vi "SeCrTS-DD signal names extracter.vi"(11 "input cluster":T1) -> (3 "Signal names":T2)   [LabVIEW 2022 SP3]
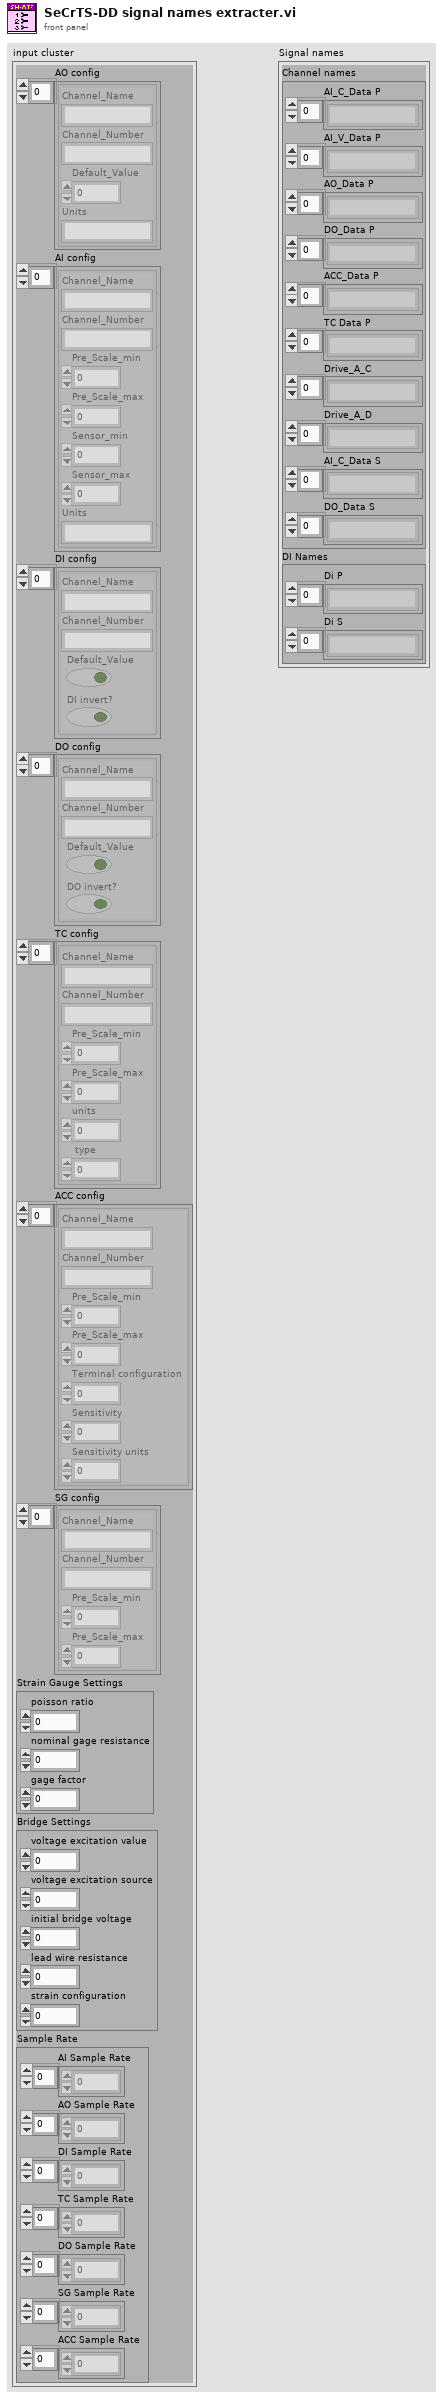
[diagram p1: front panel]
types:
  T1 = cluster{"AO config":cluster{"Channel_Name":string, "Channel_Number":string, "Default_Value":dbl, "Units":string}[], "AI config":cluster{"Channel_Name":string, "Channel_Number":string, "Pre_Scale_min":dbl, "Pre_Scale_max":dbl, "Sensor_min":dbl, "Sensor_max":dbl, "Units":string}[], "DI config":cluster{"Channel_Name":string, "Channel_Number":string, "Default_Value":bool, "DI invert?":bool}[], "DO config":cluster{"Channel_Name":string, "Channel_Number":string, "Default_Value":bool, "DO invert?":bool}[], "TC config":cluster{"Channel_Name":string, "Channel_Number":string, "Pre_Scale_min":dbl, "Pre_Scale_max":dbl, "units":i32, " type":i32}[], "ACC config":cluster{"Channel_Name":string, "Channel_Number":string, "Pre_Scale_min":dbl, "Pre_Scale_max":dbl, "Terminal configuration":i32, "Sensitivity":dbl, "Sensitivity units":i32}[], "SG config":cluster{"Channel_Name":string, "Channel_Number":string, "Pre_Scale_min":dbl, "Pre_Scale_max":dbl}[], "Strain Gauge Settings":cluster{"poisson ratio":dbl, "nominal gage resistance":dbl, "gage factor":dbl}, "Bridge Settings":cluster{"voltage excitation value":dbl, "voltage excitation source":i32, "initial bridge voltage":dbl, "lead wire resistance":dbl, "strain configuration":i32}, "Sample Rate":cluster{"AI Sample Rate":dbl[], "AO Sample Rate":dbl[], "DI Sample Rate":dbl[], "TC Sample Rate":dbl[], "DO Sample Rate":dbl[], "SG Sample Rate":dbl[], "ACC Sample Rate":dbl[]}}
  T2 = cluster{"Channel names":cluster{"AI_C_Data P":string[], "AI_V_Data P":string[], "AO_Data P":string[], "DO_Data P":string[], "ACC_Data P":string[], "TC Data P":string[], "Drive_A_C":string[], "Drive_A_D":string[], "AI_C_Data S":string[], "DO_Data S":string[]}, "DI Names":cluster{"Di P":string[], "Di S":string[]}}
  T3 = cluster{"Channel_Name":string, "Channel_Number":string, "Default_Value":dbl, "Units":string}[]
  T4 = cluster{"Channel_Name":string, "Channel_Number":string, "Pre_Scale_min":dbl, "Pre_Scale_max":dbl, "Sensor_min":dbl, "Sensor_max":dbl, "Units":string}[]
  T5 = cluster{"Channel_Name":string, "Channel_Number":string, "Default_Value":bool, "DI invert?":bool}[]
  T6 = cluster{"Channel_Name":string, "Channel_Number":string, "Default_Value":bool, "DO invert?":bool}[]
  T7 = cluster{"Channel_Name":string, "Channel_Number":string, "Pre_Scale_min":dbl, "Pre_Scale_max":dbl, "units":i32, " type":i32}[]
  T8 = cluster{"Channel_Name":string, "Channel_Number":string, "Pre_Scale_min":dbl, "Pre_Scale_max":dbl, "Terminal configuration":i32, "Sensitivity":dbl, "Sensitivity units":i32}[]
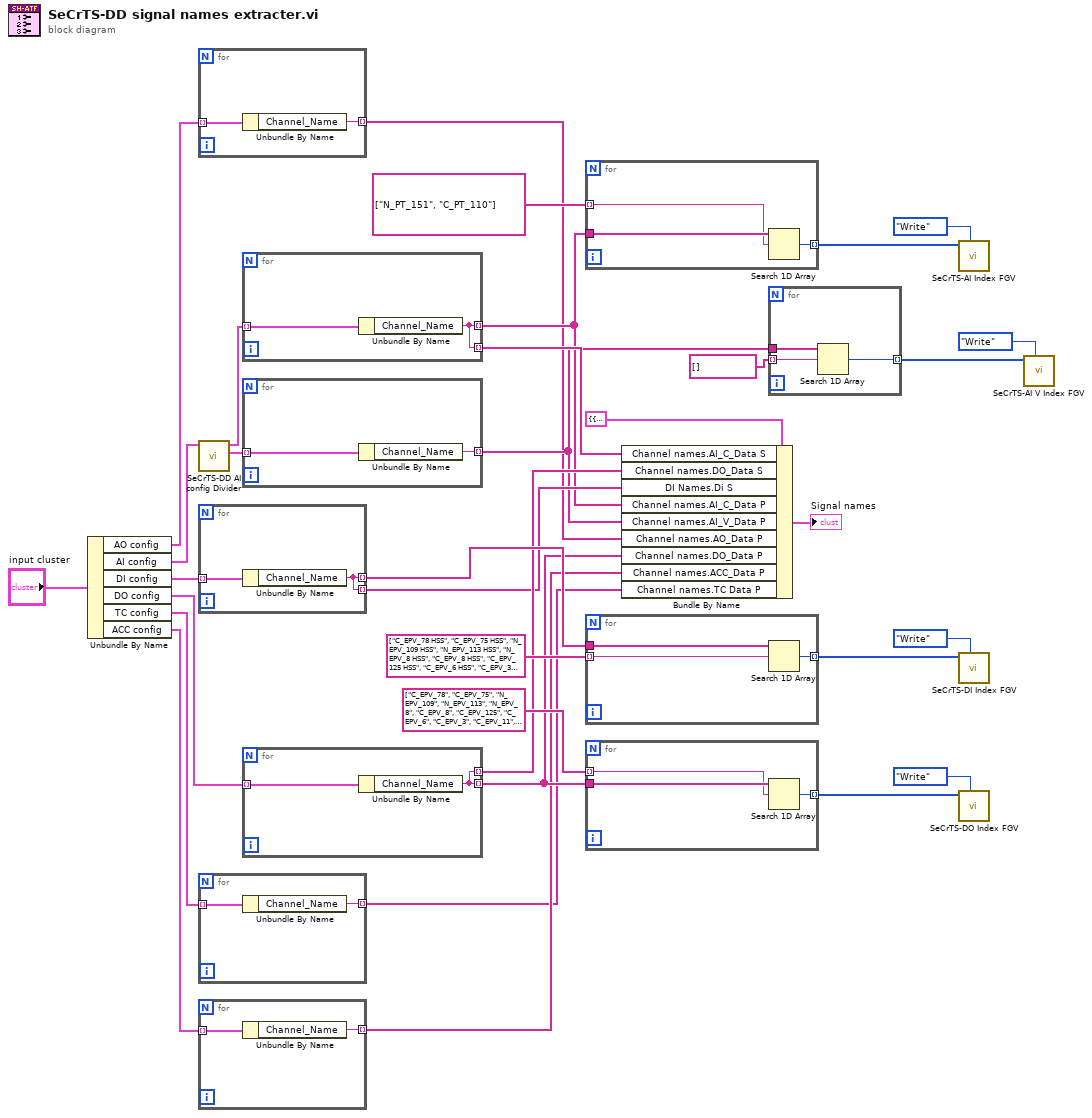
[diagram p0: block diagram]
diagram:
  n1 = Unbundle By Name("input cluster") -> ("AO config"=w25:T3, "AI config"=w30:T4, "DI config"=w26:T5, "DO config"=w27:T6, "TC config"=w28:T7, "ACC config"=w29:T8)
  n2 = for {
    tunnel: w25 -> [w35] mode=indexing
    tunnel: [w34] -> w5 mode=indexing
    n3 = Unbundle By Name(w35) -> ("Channel_Name"=w34:string)
  }
  n4 = call "SeCrTS-DD AI config Divider.vi"("AI config"=w30) -> ("AI V"=w32:T4, "AI C"=w31:T4)  [unwired: 9 in]
  n5 = for {
    tunnel: [w36] -> w14 mode=indexing
    tunnel: w26 -> [w37] mode=indexing
    tunnel: [w36] -> w8 mode=indexing
    n6 = Unbundle By Name(w37) -> ("Channel_Name"=w36:string)
  }
  n7 = for {
    tunnel: [w39] -> w2 mode=indexing
    tunnel: w28 -> [w38] mode=indexing
    n8 = Unbundle By Name(w38) -> ("Channel_Name"=w39:string)
  }
  n9 = for {
    tunnel: w29 -> [w41] mode=indexing
    tunnel: [w40] -> w3 mode=indexing
    n10 = Unbundle By Name(w41) -> ("Channel_Name"=w40:string)
  }
  n11 = for {
    tunnel: w31 -> [w43] mode=indexing
    tunnel: [w42] -> w7 mode=indexing
    tunnel: [w42] -> w10 mode=indexing
    n12 = Unbundle By Name(w43) -> ("Channel_Name"=w42:string)
  }
  n13 = for {
    tunnel: w32 -> [w45] mode=indexing
    tunnel: [w44] -> w6 mode=indexing
    n14 = Unbundle By Name(w45) -> ("Channel_Name"=w44:string)
  }
  n15 = for {
    tunnel: w27 -> [w47] mode=indexing
    tunnel: [w46] -> w4 mode=indexing
    tunnel: [w46] -> w9 mode=indexing
    n16 = Unbundle By Name(w47) -> ("Channel_Name"=w46:string)
  }
  n17 = for {
    tunnel: w7 -> [w50]
    tunnel: string[] ["N_PT_151", "C_PT_110"] ("element") -> [w49] mode=indexing
    tunnel: [w48] -> w22 mode=indexing
    n18 = Search 1D Array(1D array=w50, element=w49) -> (index of element=w48:i32)  [unwired: 1 in]
  }
  n19 = for {
    tunnel: w14 -> [w53]
    tunnel: string[] ["C_EPV_78 HSS", "C_EPV_75 HSS", "N_EPV_109 HSS", "N_EPV_113 HSS", "N_EPV_8 HSS", "C_EPV_8 HSS", "C_EPV_125 HSS", "C_EPV_6 HSS", "C_EPV_3 HSS", "C_EPV_11 HSS", "N_EPV_190 HSS", "C_EPV_14 HSS", "C_EPV_13 HSS", "N_EPV_128 HSS", "F_EPV_150 HSS", "F_EPV_41 HSS", "N_EPV_157 HSS", "F_EPV_43 HSS", "F_EPV_38 HSS", "F_EPV_45 HSS", "N_EPV_72 HSS", "F_EPV_175 HSS", "N_EPV_138 HSS", "G_EPV_69 HSS", "M_EPV_90 HSS", "N_EPV_185 HSS "] ("DI Names") -> [w52] mode=indexing
    tunnel: [w51] -> w15 mode=indexing
    n20 = Search 1D Array(1D array=w53, element=w52) -> (index of element=w51:i32)  [unwired: 1 in]
  }
  n21 = for {
    tunnel: w4 -> [w56]
    tunnel: string[] ["C_EPV_78", "C_EPV_75", "N_EPV_109", "N_EPV_113", "N_EPV_8", "C_EPV_8", "C_EPV_125", "C_EPV_6", "C_EPV_3", "C_EPV_11", "N_EPV_190", "C_EPV_14", "C_EPV_13", "N_EPV_128", "N_EPV_150", "F_EPV_41", "N_EPV_157", "F_EPV_43", "F_EPV_38", "F_EPV_45", "N_EPV_72", "F_EPV_175", "N_EPV_138", "G_EPV_69", "M_EPV_90", "N_EPV_185"] ("Array") -> [w55] mode=indexing
    tunnel: [w54] -> w18 mode=indexing
    n22 = Search 1D Array(1D array=w56, element=w55) -> (index of element=w54:i32)  [unwired: 1 in]
  }
  n23 = Bundle By Name(cluster=T2 {"Channel names"={"AI_C_Data P"=[], "AI_V_Data P"=[], "AO_Data P"=[], "DO_Data P"=[], "ACC_Data P"=[], "TC Data P"=[], "Drive_A_C"=[], "Drive_A_D"=[], "AI_C_Data S"=[], "DO_Data S"=[]}, "DI Names"={"Di P"=[], "Di S"=[]}} ("Signal names"), "Channel names.AI_C_Data S"=w10, "Channel names.DO_Data S"=w9, "DI Names.Di S"=w8, "Channel names.AI_C_Data P"=w7, "Channel names.AI_V_Data P"=w6, "Channel names.AO_Data P"=w5, "Channel names.DO_Data P"=w4, "Channel names.ACC_Data P"=w3, "Channel names.TC Data P"=w2) -> (→"Signal names":T2)
  n24 = for {
    tunnel: w6 -> [w59]
    tunnel: string[] [] ("element") -> [w58] mode=indexing
    tunnel: [w57] -> w19 mode=indexing
    n25 = Search 1D Array(1D array=w59, element=w58) -> (index of element=w57:i32)  [unwired: 1 in]
  }
  n26 = call "SeCrTS-AI Index FGV.vi"("Action"=enum16{"Write", "Read", "Init"}."Write", "Ai Index Element"=w22) -> ()  [unwired: 9 in, 1 out]
  n27 = call "SeCrTS-DI Index FGV .vi"("Action"=enum16{"Write", "Read", "Init"}."Write", "Ai Index Element"=w15) -> ()  [unwired: 9 in, 1 out]
  n28 = call "SeCrTS-DO Index FGV.vi"("Action"=enum16{"Write", "Read", "Init"}."Write", "Ai Index Element"=w18) -> ()  [unwired: 9 in, 1 out]
  n29 = call "SeCrTS-AI V Index FGV .vi"("Action"=enum16{"Write", "Read", "Init"}."Write", "Ai Index Element"=w19) -> ()  [unwired: 9 in, 1 out]
